vi "deleteEndLine (SubVI).vi"(11 "read buffer":string) -> (3 "result string":string)   [LabVIEW 2015]
doc: "Deletes \"\\r\\n\" - end of line."
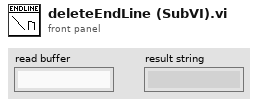
[diagram p1: front panel]
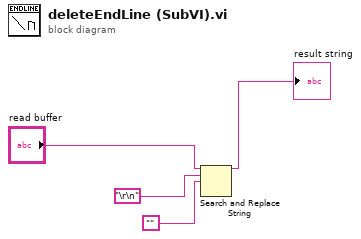
[diagram p0: block diagram]
diagram:
  n1 = Search and Replace String(input string="read buffer", search string="\r\n", replace string="") -> (result string=→"result string":string)  [unwired: 5 in, 3 out]
